vi "Run Test.vi"(8 "error in (no error)":errorcluster, 11 "Example Test In":refnum<class "Program RF MTS.lvclass">) -> (0 "error out":errorcluster, 1 "Fail Codes":string[](array[string]), 2 "Tests Passed":bool[](array[boolean]), 3 "Example Test Out":refnum<class "Program RF MTS.lvclass">)   [LabVIEW 2015]
uses:
  Test Class/Test Class.lvclass
  Classes/Application/Class/Application.lvclass
  Program App/Program RF.lvclass
  <vilib>/Cree, Inc/Cree Test Framework/Classes/Base Objects/Base Class/Base Class/Base Class.lvclass
  Program RF MTS.lvclass
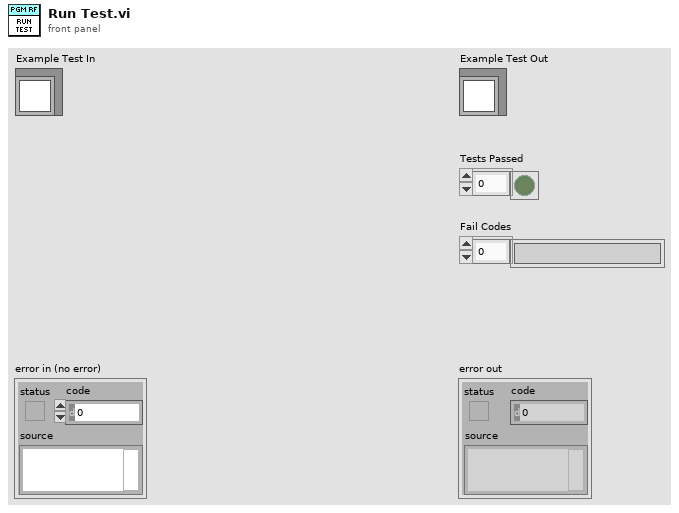
[diagram p1: front panel]
types:
  T1 = enum16{"Trace", "Debug", "Info", "Warn", "Error", "Fatal"}
  T2 = cluster{"Serial Number Reference":refnum<vi>, "Status Message Reference":refnum<vi>, "Position":u32}[]
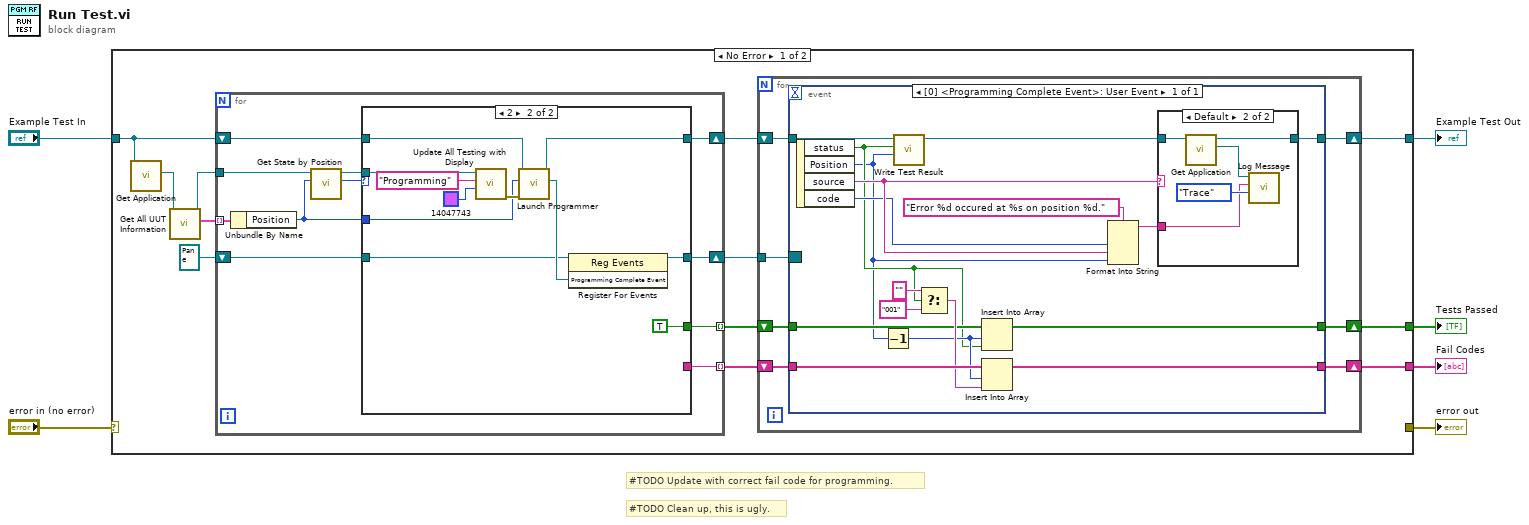
[diagram p0: block diagram]
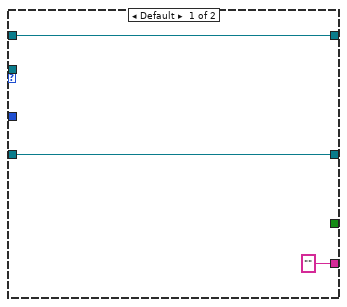
[diagram p3: hidden frame]
diagram:
  # "#TODO Clean up, this is ugly."
  # "#TODO Update with correct fail code for programming."
  n1 = case shown="No Error" "error in (no error)" {
    selector: "error in (no error)" -> [_ w75]
    tunnel: [_ w75] -> w6
    tunnel: "Example Test In" -> [w7 w74]
    tunnel: [w10 w74] -> w5
    tunnel: [w9 _] -> w2
    tunnel: [w8 _] -> w1
    frame No Error {
      n2 = call "Get Application.vi"("Test Class in"=w7) -> ("Application.lvlib:Application.lvclass"=w18:refnum<class "Application.lvclass">)  [unwired: 8 in, 2 out]
      n3 = call-dynamic "Get All UUT Information.vi"("Application in"=w18) -> ("Active UUTs"=w16:T2, "Application out"=w17:refnum<class "Application.lvclass">)  [unwired: 8 in, 1 out]
      n4 = for {
        shift-right: [w54] -> w14
        shift-left: w7 -> [w56]
        tunnel: w16 -> [w59] mode=indexing
        tunnel: w17 -> [w53]
        shift-right: [w51] -> w13
        shift-left: refnum<event-registration> refnum ("Event Registration Refnum") -> [w52]
        tunnel: [w50] -> w12 mode=indexing
        tunnel: [w49] -> w11 mode=indexing
        n5 = Unbundle By Name(w59) -> ("Position"=w55:u32)
        n6 = call-dynamic "Get State by Position.vi"("Position"=w55, "Application in"=w53) -> ("State"=w58:u32, "Application out"=w57:refnum<class "Application.lvclass">)  [unwired: 7 in, 1 out]
        n7 = case shown="2" w58 {
          tunnel: w56 -> [w62 w73]
          tunnel: [w62 w72] -> w54
          tunnel: w55 -> [_ w67]
          tunnel: w57 -> [_ w69]
          tunnel: w52 -> [w61 w64]
          tunnel: [w61 w65] -> w51
          tunnel: [_ TRUE] -> w50
          tunnel: ["" _] -> w49
          frame Default {
          }
          frame 2 {
            n8 = call "Update All Testing with Display.vi"("BG Color"=u32 14047743, "Message ('')"="Programming", "Application in"=w69) -> ("error out"=w68:errorcluster)  [unwired: 7 in, 1 out]
            n9 = call "Launch Programmer.vi"("error in (no error)"=w68, "Position"=w67, "Program RF in"=w73) -> ("Programming Complete Event"=w66:refnum<user-event>, "Program RF out"=w72:refnum<class "Program RF MTS.lvclass">)  [unwired: 6 in, 1 out]
            n10 = register-events(reference=w64, w66) -> (reference out=w65:refnum<event-registration>)  [unwired: 1 in, 1 out]
          }
        }
      }
      n11 = for {
        shift-right: [w23] -> w10
        shift-left: w14 -> [w25]
        tunnel: w13 -> [w24]
        shift-right: [w20] -> w9
        shift-left: w12 -> [w22]
        shift-right: [w19] -> w8
        shift-left: w11 -> [w21]
        n12 = event shown="[0] <Programming Complete Event>: User Event" {
          selector: w24 -> [_]
          dyn-events: _ -> [_]
          timeout: _ -> [_]
          tunnel: w25 -> [w40]
          tunnel: [w38] -> w23
          tunnel: w22 -> [w32]
          tunnel: w21 -> [w34]
          tunnel: [w29] -> w20
          tunnel: [w28] -> w19
          event User Event {
            n13 = event-data() -> ("status"=w30:bool, "Position"=w27:u32, "source"=w36:string, "code"=w35:i32)  [unwired: 1 in]
            n14 = Decrement(x=w27) -> (x-1=w31:u32)
            n15 = call "Write Test Result.vi"("Position"=w27, "Test Passed"=w30, "Test Class.lvclass"=w40) -> ("Test Class.lvclass"=w39:refnum<class "Program RF MTS.lvclass">)  [unwired: 7 in, 1 out]
            n16 = Select(t="", s=w30, f="001") -> (s? t:f=w33:string)
            n17 = Insert Into Array(array=w32, index=w31, new element=w30) -> (w29:bool[])
            n18 = Insert Into Array(array=w34, index=w31, new element=w33) -> (w28:string[])
            n19 = Format Into String(format string="Error %d occured at %s on position %d.", w35, w36, w27) -> (resulting string=w37:string)  [unwired: 2 in, 1 out]
            n20 = case shown="Default" w36 {
              tunnel: w39 -> [w43 w47]
              tunnel: [w43 w46] -> w38
              tunnel: w37 -> [_ w44]
              frame "" {
              }
              frame Default {
                n21 = call "Get Application.vi"("Test Class in"=w47) -> ("Application.lvlib:Application.lvclass"=w48:refnum<class "Application.lvclass">, "Test Class out"=w46:refnum<class "Program RF MTS.lvclass">)  [unwired: 8 in, 1 out]
                n22 = call <vilib>:"Log Message.vi"("Level"=T1."Trace", "Event"=w44, "Base Class in"=w48) -> ()  [unwired: 7 in, 2 out]
              }
            }
          }
        }
      }
    }
    frame Error {
    }
  }
  "error out" <- w6
  "Example Test Out" <- w5
  "Tests Passed" <- w2
  "Fail Codes" <- w1
